vi "Register by Name.vi"(6 "Get Last Broadcast Event (F)":bool, 7 "Event":refnum<class "Event.lvclass">, 8 "error in (no error)":errorcluster, 9 "Event Fire Handler":refnum<class "Abstract Event Message for View.lvclass">, 10 "View Name":string, 11 "Controller in":refnum<class "Controller.lvclass">) -> (0 "error out":errorcluster, 3 "Controller out":refnum<class "Controller.lvclass">)   [LabVIEW 2023, in "MVC Actors.lvlib" / "Controller.lvclass"]
doc: "Lets a View specified by <b>View Name</b> register an <b>Event</b> to the Controller by providing an <b>Event Handler</b>."
uses:
  Controller.lvclass
  Event/Event.lvclass
  Event Handlers/Abstract Event Message for View/Abstract Event Message for View.lvclass
  Controller.lvclass/Controller.ctl
  View Details.ctl
  <vilib>/ActorFramework/Message Enqueuer/Message Enqueuer.lvclass
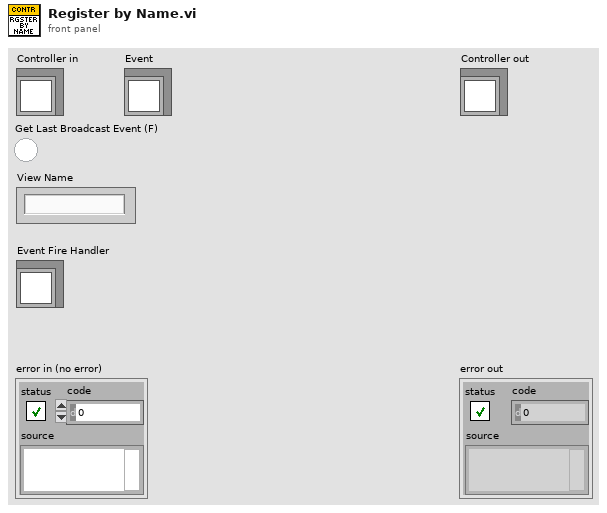
[diagram p1: front panel]
types:
  T1 = typedef "MVC Actors.lvlib/Controller.lvclass/View Details.ctl" = cluster{"Exclude From Broadcast":bool, "Receive Only":bool, "Paused":bool, "View Enqueuer":refnum<class "Message Enqueuer.lvclass">}
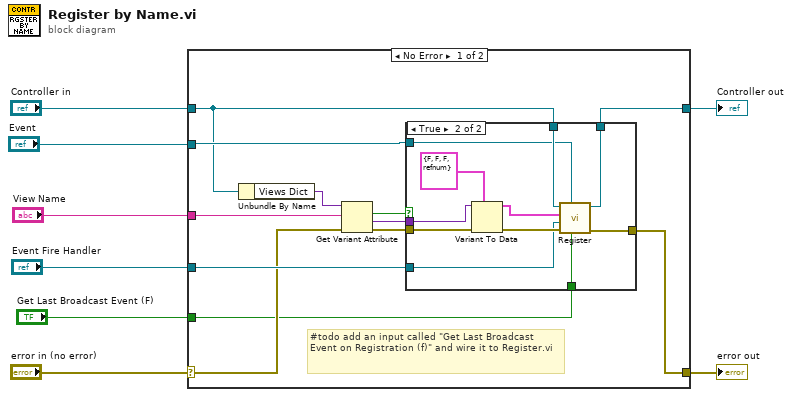
[diagram p0: block diagram]
diagram:
  n1 = case shown="No Error" "error in (no error)" {
    selector: "error in (no error)" -> [w11 w35]
    tunnel: [w10 w35] -> w7
    tunnel: [w12 w34] -> w5
    tunnel: "Controller in" -> [w13 w34]
    tunnel: "View Name" -> [w19 _]
    tunnel: "Event Fire Handler" -> [w15 _]
    tunnel: "Event" -> [w14 _]
    tunnel: "Get Last Broadcast Event (F)" -> [w9 _]
    frame No Error {
      # "#todo add an input called \"Get Last Broadcast Event on Registration (f)\" and wire it to Register.vi"
      n2 = Unbundle By Name(w13) -> ("Views Dict"=w20:variant)
      n3 = Get Variant Attribute(Variant=w20, name=w19, error in=w11) -> (found=w18:bool, value=w17:variant, error out=w16:errorcluster)  [unwired: 1 in, 1 out]
      n4 = case shown="True" w18 {
        tunnel: w17 -> [_ w32]
        tunnel: w16 -> [w22 w33]
        tunnel: w15 -> [_ w30]
        tunnel: w13 -> [w21 w29]
        tunnel: w14 -> [_ w28]
        tunnel: [w22 w27] -> w10
        tunnel: [w21 w26] -> w12
        tunnel: w9 -> [_ w23]
        frame False {
        }
        frame True {
          n5 = Variant To Data(error in=w33, type=T1 {"Exclude From Broadcast"=FALSE, "Receive Only"=FALSE, "Paused"=FALSE, "View Enqueuer"=refnum} ("Message Enqueuer"), Variant=w32) -> (data=w24:T1, error out=w31:errorcluster)
          n6 = call "Register.vi"("Get Last Broadcast Event (F)"=w23, "Event"=w28, "Error In"=w31, "View Event Fire Handler"=w30, "Registrant Details"=w24, "Controller Actor In"=w29) -> ("Error Out"=w27:errorcluster, "Controller Actor Out"=w26:refnum<class "Controller.lvclass">)  [unwired: 4 in]
        }
      }
    }
    frame Error {
    }
  }
  "error out" <- w7
  "Controller out" <- w5
